vi "Write condtional.vi"(5 "condtional":bool, 9 "ForLoop in":refnum<class "WhileLoop.lvclass">) -> (3 "ForLoop out":refnum<class "WhileLoop.lvclass">)   [LabVIEW 2014]
uses:
  WhileLoop.lvclass
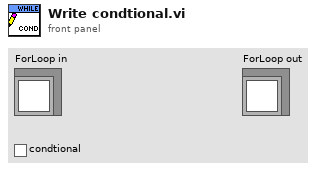
[diagram p1: front panel]
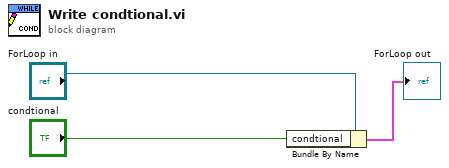
[diagram p0: block diagram]
diagram:
  n1 = Bundle By Name(cluster="ForLoop in", "condtional"="condtional") -> (→"ForLoop out":cluster{})
